vi "RefToArray.vi"(1 "ArrayRef":refnum<vi>) -> (0 "Array":cluster{"TestStep":string[], "Enable":bool[]}[](array[cluster]))   [LabVIEW 2009]
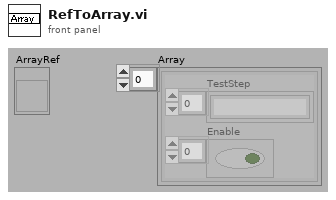
[diagram p1: front panel]
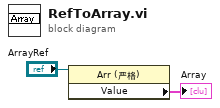
[diagram p0: block diagram]
diagram:
  n1 = property class="Arr (严格)"(reference="ArrayRef") -> ("Value"=→"Array":cluster{"TestStep":string[], "Enable":bool[]}[])  [unwired: 1 in, 2 out]
